vi "24-1.vi"() -> ()   [LabVIEW 2019, in "24.lvlib"]
uses:
  24.lvlib
panel:
  in  "Sample?":bool
  out "Largest Vailid":u8[](array[numeric])
  in  "Sample Index":i32
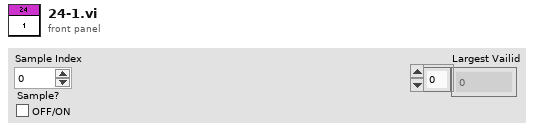
[diagram p1: front panel]
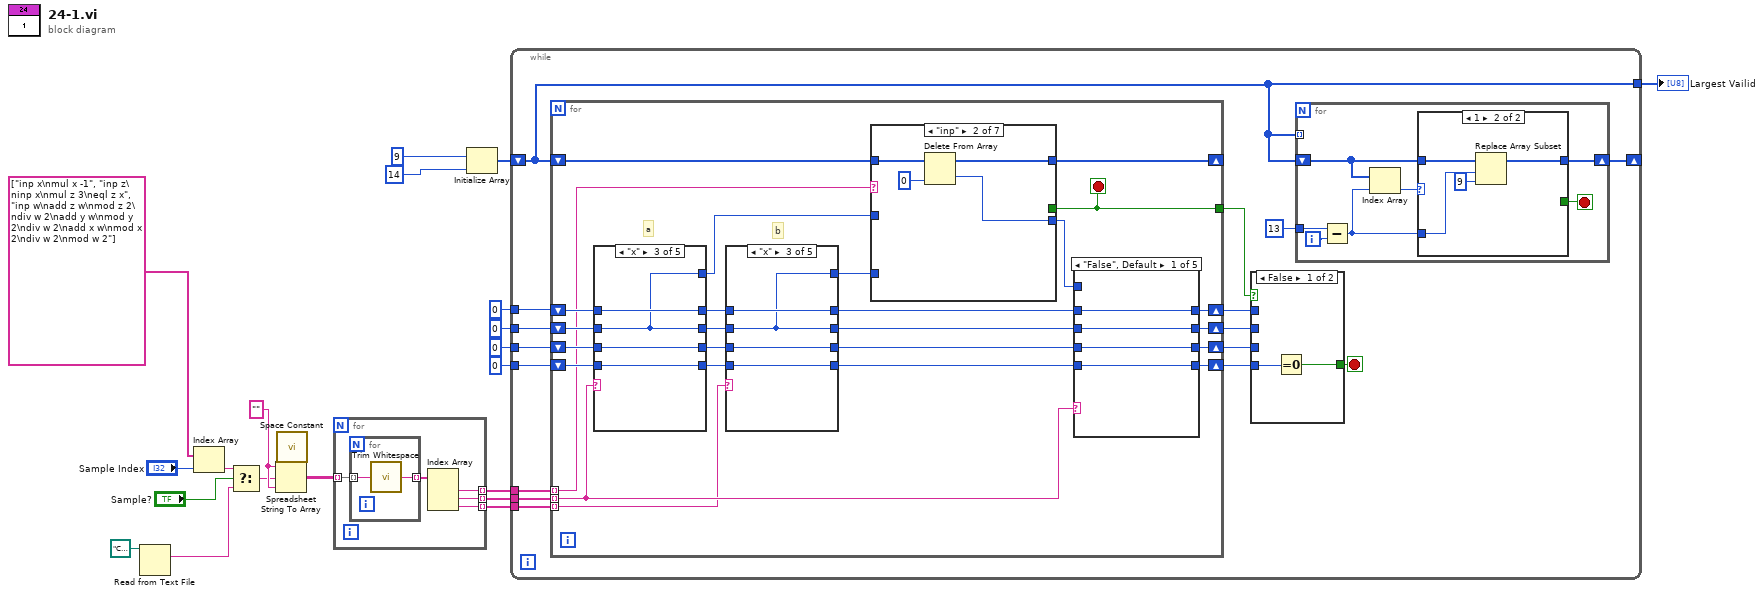
[diagram p0: block diagram]
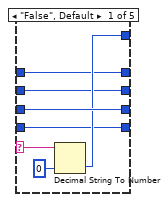
[diagram p2: hidden frame]
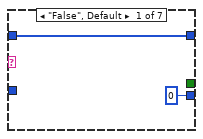
[diagram p10: hidden frame]
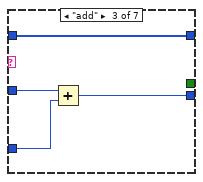
[diagram p11: hidden frame]
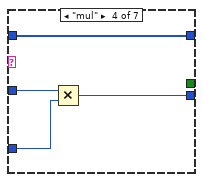
[diagram p12: hidden frame]
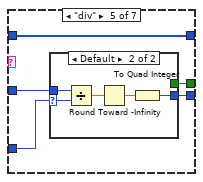
[diagram p13: hidden frame]
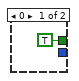
[diagram p14: hidden frame]
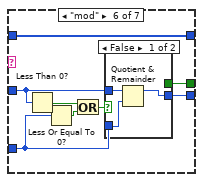
[diagram p15: hidden frame]
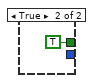
[diagram p16: hidden frame]
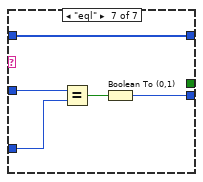
[diagram p17: hidden frame]
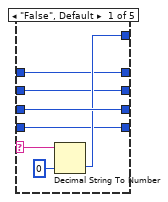
[diagram p18: hidden frame]
diagram:
  w19 = "" ("format string")
  n1 = Read from Text File(file (use dialog)=path "C:/Users/craig.walker/Documents/GitHub/lv2019-Advent-of-Code-2021/24/input.txt") -> (text=w10:string)  [unwired: 3 in, 3 out]
  n2 = Index Array(array=string[] ["inp x\nmul x -1", "inp z\ninp x\nmul z 3\neql z x", "inp w\nadd z w\nmod z 2\ndiv w 2\nadd y w\nmod y 2\ndiv w 2\nadd x w\nmod x 2\ndiv w 2\nmod w 2"] ("format string"), index="Sample Index") -> (element=w11:string)
  n3 = Select(t=w11, s="Sample?", f=w10) -> (s? t:f=w12:string)
  n4 = call <vilib>:"Space Constant.vi"() -> ("String"=w18:string)
  n5 = Spreadsheet String To Array(delimiter (Tab)=w18, format string=w19, spreadsheet string=w12, array type (2D Dbl)=w19) -> (array=w13:string[][])
  n6 = for {
    tunnel: w13 -> [w26] mode=indexing
    tunnel: [w24] -> w3 mode=indexing
    tunnel: [w23] -> w2 mode=indexing
    tunnel: [w22] -> w1 mode=indexing
    n7 = for {
      tunnel: [w27] -> w25 mode=indexing
      tunnel: w26 -> [w28] mode=indexing
      n8 = call <vilib>:"Trim Whitespace.vi"("string"=w28) -> ("trimmed string"=w27:string)  [unwired: 1 in]
    }
    n9 = Index Array(array=w25) -> (element #1=w24:string, element #2=w23:string, element #3=w22:string)  [unwired: 3 in]
  }
  n10 = Initialize Array(u8 9 ("element"), 14 ("dimension size")) -> (w15:u8[])
  n11 = while {
    tunnel: [w41] -> w14
    shift-right: [w42] -> _
    shift-left: w15 -> [w41]
    tunnel: i64 0 ("w") -> [w39]
    tunnel: i64 0 ("x") -> [w38]
    tunnel: i64 0 ("y") -> [w37]
    tunnel: i64 0 ("z") -> [w36]
    tunnel: w3 -> [w34]
    tunnel: w2 -> [w33]
    tunnel: w1 -> [w32]
    stop <- w44 stop-if-true
    n12 = for {
      shift-right: [w68] -> w29
      shift-left: w37 -> [w69]
      shift-right: [w64] -> _
      shift-left: w41 -> [w65]
      tunnel: [w63] -> w40
      shift-right: [w48] -> w31
      shift-left: w39 -> [w62]
      shift-right: [w49] -> w30
      shift-left: w38 -> [w61]
      shift-right: [w50] -> w35
      shift-left: w36 -> [w60]
      tunnel: w34 -> [w47] mode=indexing
      tunnel: w33 -> [w46] mode=indexing
      tunnel: w32 -> [w45] mode=indexing
      stop <- w63 stop-if-true
      # "b"
      # "a"
      n13 = case shown="\"x\"" w46 {
        selector: w46 -> [w160 _ _ _ _]
        tunnel: w69 -> [w161 w163 w167 w170 w177]
        tunnel: [w161 w163 w167 w170 w177] -> w56
        tunnel: [w158 w164 w166 w170 w174] -> w67
        tunnel: w62 -> [w156 w164 w169 w173 w175]
        tunnel: w61 -> [w157 w165 w166 w172 w176]
        tunnel: w60 -> [w155 w162 w168 w171 w174]
        tunnel: [w156 w164 w169 w173 w175] -> w59
        tunnel: [w157 w165 w166 w172 w176] -> w55
        tunnel: [w155 w162 w168 w171 w174] -> w57
        frame "False", Default {
          n14 = Decimal String To Number(string=w160, default (0L)=i64 0 ("default (0 I32)")) -> (number=w158:i64)  [unwired: 1 in, 1 out]
        }
        frame "w" {
        }
        frame "x" {
        }
        frame "y" {
        }
        frame "z" {
        }
      }
      n15 = case shown="\"x\"" w45 {
        selector: w45 -> [w75 _ _ _ _]
        tunnel: w56 -> [w76 w78 w82 w85 w92]
        tunnel: [w76 w78 w82 w85 w92] -> w54
        tunnel: [w73 w79 w81 w85 w89] -> w58
        tunnel: w59 -> [w71 w79 w84 w88 w90]
        tunnel: w55 -> [w72 w80 w81 w87 w91]
        tunnel: w57 -> [w70 w77 w83 w86 w89]
        tunnel: [w71 w79 w84 w88 w90] -> w52
        tunnel: [w72 w80 w81 w87 w91] -> w53
        tunnel: [w70 w77 w83 w86 w89] -> w51
        frame "False", Default {
          n16 = Decimal String To Number(string=w75, default (0L)=i64 0 ("default (0 I32)")) -> (number=w73:i64)  [unwired: 1 in, 1 out]
        }
        frame "w" {
        }
        frame "x" {
        }
        frame "y" {
        }
        frame "z" {
        }
      }
      n17 = case shown="\"inp\"" w47 {
        tunnel: w67 -> [_ _ w121 w125 w130 w143 w153]
        tunnel: w58 -> [_ _ w120 w124 w129 w142 w152]
        tunnel: [i64 0 ("z") w115 w119 w123 w128 w144 w150] -> w66
        tunnel: w65 -> [w113 w118 w122 w126 w131 w145 w154]
        tunnel: [w113 w116 w122 w126 w131 w145 w154] -> w64
        tunnel: [_ _ _ _ w127 w138 _] -> w63
        frame "False", Default {
        }
        frame "inp" {
          n18 = Delete From Array(array=w118, index=0) -> (deleted portion=w115:u8, array with subset deleted=w116:u8[])  [unwired: 1 in]
        }
        frame "add" {
          n19 = Add(x=w121, y=w120) -> (x+y=w119:i64)
        }
        frame "mul" {
          n20 = Multiply(x=w125, y=w124) -> (x*y=w123:i64)
        }
        frame "div" {
          n21 = case shown="Default" w129 {
            selector: w129 -> [_ w136]
            tunnel: w130 -> [_ w137]
            tunnel: [_ w133] -> w128
            tunnel: [TRUE _] -> w127
            frame 0 {
            }
            frame Default {
              n22 = Divide(x=w137, y=w136) -> (x/y=w135:dbl)
              n23 = Round Toward -Infinity(1:w135) -> (0:w134:dbl)
              n24 = To Quad Integer(1:w134) -> (0:w133:i64)
            }
          }
        }
        frame "mod" {
          n25 = Less Than 0?(x=w143) -> (x < 0?=w141:bool)
          n26 = Less Or Equal To 0?(x=w142) -> (x <= 0?=w140:bool)
          n27 = Or(x=w141, y=w140) -> (x .or. y?=w139:bool)
          n28 = case shown="False" w139 {
            tunnel: [w148 _] -> w144
            tunnel: w143 -> [w147 _]
            tunnel: w142 -> [w146 _]
            tunnel: [_ TRUE] -> w138
            frame False {
              n29 = Quotient & Remainder(x=w147, y=w146) -> (x-y*floor(x/y)=w148:i64)  [unwired: 1 out]
            }
            frame True {
            }
          }
        }
        frame "eql" {
          n30 = Equal?(x=w153, y=w152) -> (x = y?=w151:bool)
          n31 = Boolean To (0,1)(Boolean=w151) -> (0, 1=w150:i16)
        }
      }
      n32 = case shown="\"False\", Default" w46 {
        tunnel: w54 -> [w96 w98 w102 _ w109]
        tunnel: [w96 w98 w102 w105 w109] -> w68
        tunnel: w66 -> [_ w100 w103 w105 w111]
        tunnel: w53 -> [w94 w99 _ w107 w110]
        tunnel: w52 -> [w95 _ w104 w108 w112]
        tunnel: w51 -> [w93 w97 w101 w106 _]
        tunnel: [w95 w100 w104 w108 w112] -> w48
        tunnel: [w93 w97 w101 w106 w111] -> w50
        tunnel: [w94 w99 w103 w107 w110] -> w49
        frame "False", Default {
        }
        frame "w" {
        }
        frame "x" {
        }
        frame "y" {
        }
        frame "z" {
        }
      }
    }
    n33 = case shown="False" w40 {
      tunnel: w35 -> [w178 _]
      tunnel: [w179 _] -> w44
      tunnel: w31 -> [_ _]
      tunnel: w30 -> [_ _]
      tunnel: w29 -> [_ _]
      frame False {
        n34 = Equal To 0?(x=w178) -> (x = 0?=w179:bool)
      }
      frame True {
      }
    }
    n35 = for {
      tunnel: 13 ("dimension size") -> [w186]
      shift-right: [w181] -> w42
      shift-left: w41 -> [w183]
      tunnel: w41 -> [_] mode=indexing
      i -> [w185]
      stop <- w180 stop-if-true
      n36 = Subtract(x=w186, y=w185) -> (x-y=w182:i32)
      n37 = Index Array(array=w183, index=w182) -> (element=w184:u8)
      n38 = case shown="1" w184 {
        selector: w184 -> [w192 _]
        tunnel: w183 -> [w191 w196]
        tunnel: w182 -> [w189 w193]
        tunnel: [w188 w195] -> w181
        tunnel: [TRUE _] -> w180
        frame Default {
          n39 = Decrement(x=w192) -> (x-1=w190:u8)
          n40 = Replace Array Subset(array=w191, new element=w190, index=w189) -> (w188:u8[])
        }
        frame 1 {
          n41 = Replace Array Subset(array=w196, new element=u8 9 ("new element/subarray"), index=w193) -> (w195:u8[])
        }
      }
    }
  }
  "Largest Vailid" <- w14
